vi "mqttCmdBuildVarHdrInternal.vi"(8 "error in (no error)":errorcluster, 9 "keepAlive(sec)":u16, 10 "connFlagByte":u8) -> (0 "error out":errorcluster, 2 "varHeader":u8[](array[numeric]) format="%x")   [LabVIEW 2020, in "ConnectMqttMsg.lvclass"]
uses:
  ConnectMqttMsg.lvclass
  BaseMqttMsg.lvclass
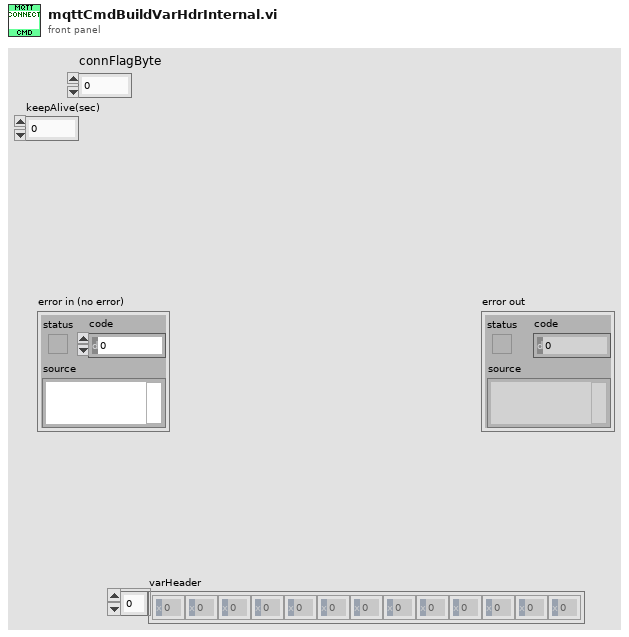
[diagram p1: front panel]
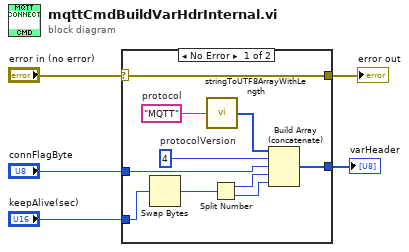
[diagram p0: block diagram]
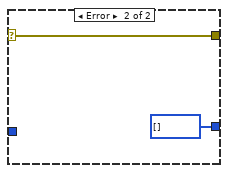
[diagram p2: hidden frame]
diagram:
  n1 = case shown="No Error" "error in (no error)" {
    selector: "error in (no error)" -> [w15 w17]
    tunnel: [w15 w17] -> w4
    tunnel: "connFlagByte" -> [w8 _]
    tunnel: "keepAlive(sec)" -> [w7 _]
    tunnel: [w6 u8[] []] -> w2
    frame No Error {
      w11 = u8 4  # protocolVersion
      w10 = "MQTT"  # protocol
      n2 = Swap Bytes(anything=w7) -> (byte swapped=w14:u16)
      n3 = call "stringToUTF8ArrayWithLength.vi"("string"=w10) -> ("UTF8[]"=w9:u8[])  [unwired: 14 in]
      n4 = Split Number(x=w14) -> (hi(x)=w13:u8, lo(x)=w12:u8)
      n5 = Build Array (concatenate)(w9, w11, w8, w13, w12) -> (w6:u8[])
    }
    frame Error {
    }
  }
  "error out" <- w4
  "varHeader" <- w2
